vi "IsGetter.vi"(8 "error in (no error)":errorcluster, 10 "vi reference":refnum<vi>) -> (0 "error out":errorcluster, 1 "IsGetter?":bool, 2 "vi reference out":refnum<vi>)   [LabVIEW 2023, in "ClassReflector.lvclass"]
uses:
  ClassReflector.lvclass
panel:
  out "VI Name":string
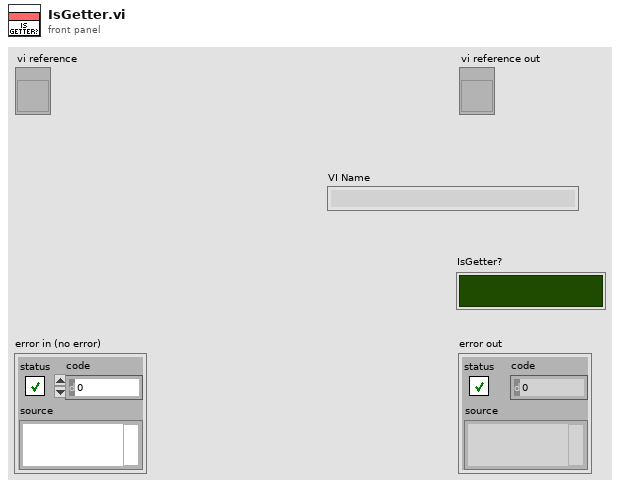
[diagram p1: front panel]
types:
  T1 = enum32{"Bad", "Idle", "Run top level", "Running"}
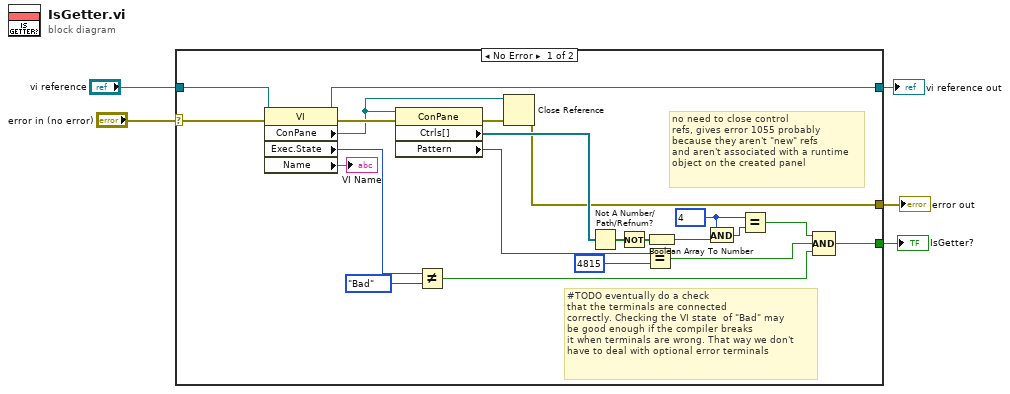
[diagram p0: block diagram]
diagram:
  n1 = case shown="No Error" "error in (no error)" {
    selector: "error in (no error)" -> [w17 w29]
    tunnel: [w14 w29] -> w4
    tunnel: [w19 _] -> w3
    tunnel: "vi reference" -> [w16 w28]
    tunnel: [w15 w28] -> w1
    frame No Error {
      w12 = u32 4 ("x")
      # "no need to close control\nrefs, gives error 1055 probably\nbecause they aren't \"new\" refs\nand aren't associated with a runtime\nobject on the created panel"
      # "#TODO eventually do a check\nthat the terminals are connected\ncorrectly. Checking the VI state  of \"Bad\" may\nbe good enough if the compiler breaks\nit when terminals are wrong. That way we don't\nhave to deal with optional error terminals"
      n2 = property class="VI"(reference=w16, error in=w17) -> (reference out=w15:refnum<vi>, error out=w27:errorcluster, "ConPane"=w26:refnum<vi>, "Exec.State"=w22:T1, "Name"=→"VI Name":string)
      n3 = property class="ConPane"(reference=w26, error in=w27) -> (error out=w13:errorcluster, "Ctrls[]"=w18:refnum<vi>[], "Pattern"=w25:u32)  [unwired: 1 out]
      n4 = Not Equal?(x=w22, y=T1."Bad") -> (x != y?=w20:bool)
      n5 = Close Reference(reference=w26, error in (no error)=w13) -> (error out=w14:errorcluster)
      n6 = Not A Number/Path/Refnum?(number/path/refnum=w18) -> (NaN/Path/Refnum?=w8:bool[])
      n7 = Not(x=w8) -> (.not. x?=w6:bool[])
      n8 = Equal?(x=w25, y=u32 4815) -> (x = y?=w23:bool)
      n9 = Boolean Array To Number(Boolean array=w6) -> (number=w7:u32)
      n10 = And(x=w12, y=w7) -> (x .and. y?=w11:u32)
      n11 = Equal?(x=w12, y=w11) -> (x = y?=w10:bool)
      n12 = Compound Arithmetic op=AND(w10, w23, w20) -> (w19:bool)
    }
    frame Error {
    }
  }
  "error out" <- w4
  "IsGetter?" <- w3
  "vi reference out" <- w1
